vi "Get or Add SharedStringTable.vi"(8 "error in":errorcluster, 11 "SharedStringTablePart in":refnum<k24>) -> (0 "error out":errorcluster, 2 "SharedStringTable":refnum<k24>, 3 "SharedStringTablePart out":refnum<k24>)   [LabVIEW 2021, in "Open Xml.lvlib"]
uses:
  Open Xml.lvlib
  D:/git/Open-Xml-LabVIEW/dll/DocumentFormat.OpenXml.dll
  dll/DocumentFormat.OpenXml.dll
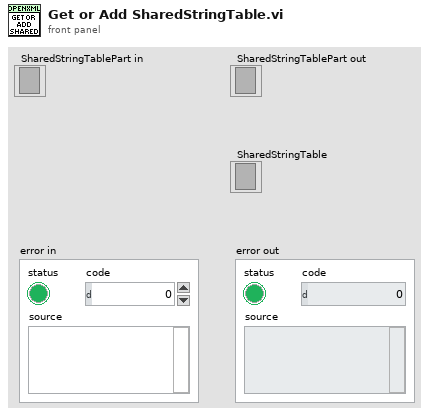
[diagram p1: front panel]
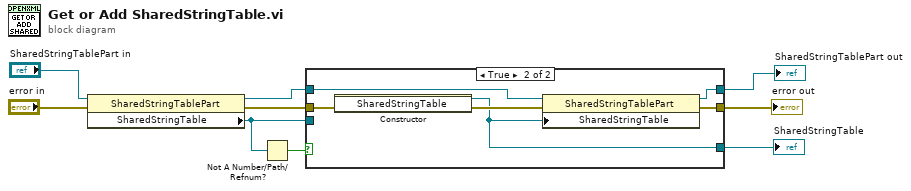
[diagram p0: block diagram]
diagram:
  n1 = property class="SharedStringTablePart"(reference="SharedStringTablePart in", error in="error in") -> (reference out=w5:refnum<k24>, error out=w7:errorcluster, "SharedStringTable"=w1:refnum<k24>)
  n2 = Not A Number/Path/Refnum?(number/path/refnum=w1) -> (NaN/Path/Refnum?=w3:bool)
  n3 = case shown="True" w3 {
    tunnel: w7 -> [w10 w18]
    tunnel: [w10 w16] -> w6
    tunnel: w5 -> [w11 w15]
    tunnel: [w11 w14] -> w4
    tunnel: [w12 w13] -> w2
    tunnel: w1 -> [w12 _]
    frame False {
    }
    frame True {
      n4 = constructor class="SharedStringTable"(error in=w18) -> (reference out=w13:refnum<k24>, error out=w17:errorcluster)  [unwired: 2 in, 1 out]
      n5 = property class="SharedStringTablePart"(reference=w15, error in=w17, "SharedStringTable"=w13) -> (reference out=w14:refnum<k24>, error out=w16:errorcluster)
    }
  }
  "SharedStringTablePart out" <- w4
  "error out" <- w6
  "SharedStringTable" <- w2
